vi "FL_Get_Speed_Histogram_Bin_number.vi"(1 "Current speed":dbl format="%#_13g", 2 "Bins array":dbl[](array[numeric])) -> (0 "Bin assignment":i32)   [LabVIEW 2016]
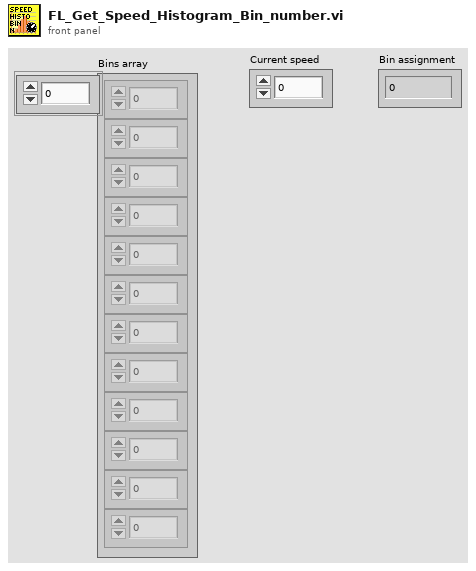
[diagram p1: front panel]
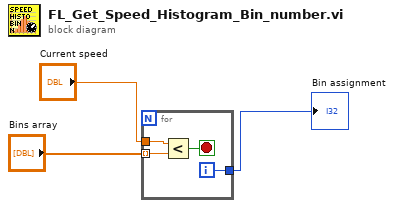
[diagram p0: block diagram]
diagram:
  n1 = for {
    tunnel: "Bins array" -> [w6] mode=indexing
    tunnel: "Current speed" -> [w7]
    tunnel: [w4] -> w1
    i -> [w4]
    stop <- w5 stop-if-true
    n2 = Less?(x=w7, y=w6) -> (x < y?=w5:bool)
  }
  "Bin assignment" <- w1
